vi "test_WFCompose.vi"() -> ()   [LabVIEW 2013]
panel:
  out "Rep4 Waveform Graph":waveform(dbl)(graph)={"t0"=timestamp(0 s since 1904-01-01), "dt"=5e-05, "Y"=array[24000 elements]}
  out "Rep3 Waveform Graph":waveform(dbl)(graph)={"t0"=timestamp(0 s since 1904-01-01), "dt"=5e-05, "Y"=array[32004 elements]}
  in  "Repetitions 4":T1={"Rep type"=3, "Duration (s)"=0.4321, "Delay (s)"=0.1234, "Interval (s)"=0.2, "M"=5} {"Rep type" items=["Off", "DC", "Trig", "Train"]}
  in  "Repetitions 3":T1={"Rep type"=3, "Duration (s)"=0.4321, "Delay (s)"=0.1234, "Interval (s)"=0.4, "M"=3} {"Rep type" items=["Off", "DC", "Trig", "Train"]}
  out "Rep2 Waveform Graph":waveform(dbl)(graph)={"t0"=timestamp(0 s since 1904-01-01), "dt"=5e-05, "Y"=array[4000 elements]}
  in  "Repetitions 2":T1={"Rep type"=2, "Duration (s)"=0.15, "Delay (s)"=0.05, "Interval (s)"=0.0, "M"=1} {"Rep type" items=["Off", "DC", "Trig", "Train"]}
  out "Rep1 Waveform Graph":waveform(dbl)(graph)={"t0"=timestamp(0 s since 1904-01-01), "dt"=5e-05, "Y"=array[12001 elements]}
  in  "Repetitions 1":T1={"Rep type"=2, "Duration (s)"=0.5, "Delay (s)"=0.1, "Interval (s)"=0.0, "M"=1} {"Rep type" items=["Off", "DC", "Trig", "Train"]}
  out "Waveform Out":waveform(dbl)={"t0"=timestamp(0 s since 1904-01-01), "dt"=5e-05, "Y"=array[4999 elements]}
  in  "Waveform Properties":T2={"Fs (Hz)"=20000.0, "Amplitude (V)"=5.0, "Ramp (s)"=0.02, "Duration (s)"=0.25} {"Ramp (s)" min=0.0; "Fs (Hz)" min=0.0}
  out "Mother Waveform Graph":waveform(dbl)(graph)={"t0"=timestamp(0 s since 1904-01-01), "dt"=5e-05, "Y"=array[4999 elements]}
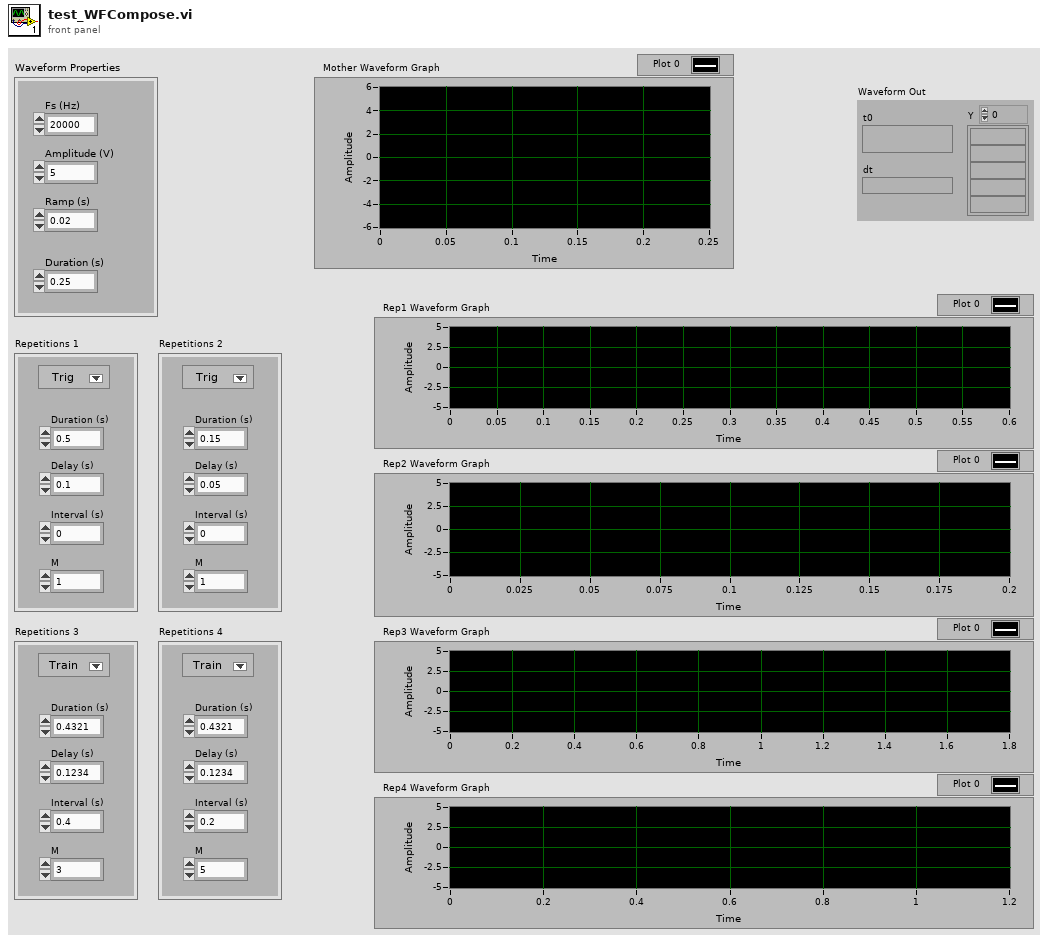
[diagram p1: front panel]
types:
  T1 = cluster{"Rep type":u16, "Duration (s)":dbl, "Delay (s)":dbl, "Interval (s)":dbl, "M":i32}
  T2 = cluster{"Fs (Hz)":dbl, "Amplitude (V)":dbl, "Ramp (s)":dbl, "Duration (s)":dbl}
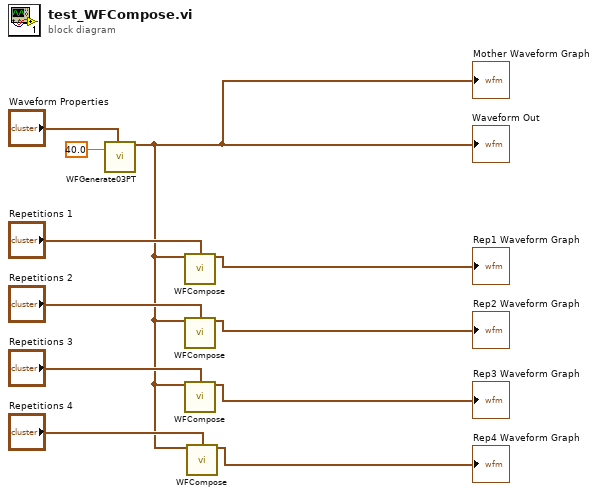
[diagram p0: block diagram]
diagram:
  n1 = call "WFGenerate03PT.vi"("Param 0"=40.0, "Waveform Properties"="Waveform Properties") -> ("Waveform Out"=w3:waveform(dbl))  [unwired: 16 in, 1 out]
  "Mother Waveform Graph" <- w3
  "Waveform Out" <- w3
  n2 = call "WFCompose.vi"("Waveform In"=w3, "Repetitions"="Repetitions 1") -> ("Analog Waveform Out"=→"Rep1 Waveform Graph":waveform(dbl))  [unwired: 11 in, 2 out]
  n3 = call "WFCompose.vi"("Waveform In"=w3, "Repetitions"="Repetitions 2") -> ("Analog Waveform Out"=→"Rep2 Waveform Graph":waveform(dbl))  [unwired: 11 in, 2 out]
  n4 = call "WFCompose.vi"("Waveform In"=w3, "Repetitions"="Repetitions 3") -> ("Analog Waveform Out"=→"Rep3 Waveform Graph":waveform(dbl))  [unwired: 11 in, 2 out]
  n5 = call "WFCompose.vi"("Waveform In"=w3, "Repetitions"="Repetitions 4") -> ("Analog Waveform Out"=→"Rep4 Waveform Graph":waveform(dbl))  [unwired: 11 in, 2 out]
